vi "Get Menus.vi"(8 "error in (no error)":errorcluster, 9 "Name":string, 10 "RightMenu":refnum<vi>, 11 "Left Menu":refnum<vi>) -> (0 "error out":errorcluster)   [LabVIEW 2020]
doc: "This VI provides access to the defined set of menus, returning whichever is requested by the caller. It provides encapsulation of the menu list, so the list can be updated/modified without having to change this function or its callers."
uses:
  Controls/Menu.ctl
  Controls/Menus.ctl
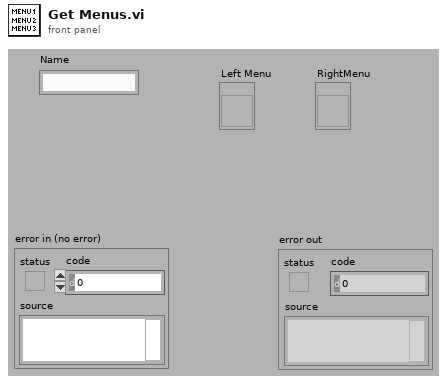
[diagram p1: front panel]
types:
  T1 = typedef "Menus.ctl" = cluster{"Menu Name":string, "Left Menu":T2, "Right Menu":T2}[]
  T2 = typedef "Menu.ctl" = cluster{"Menu 0":string, "Menu 1":string, "Menu 2":string}
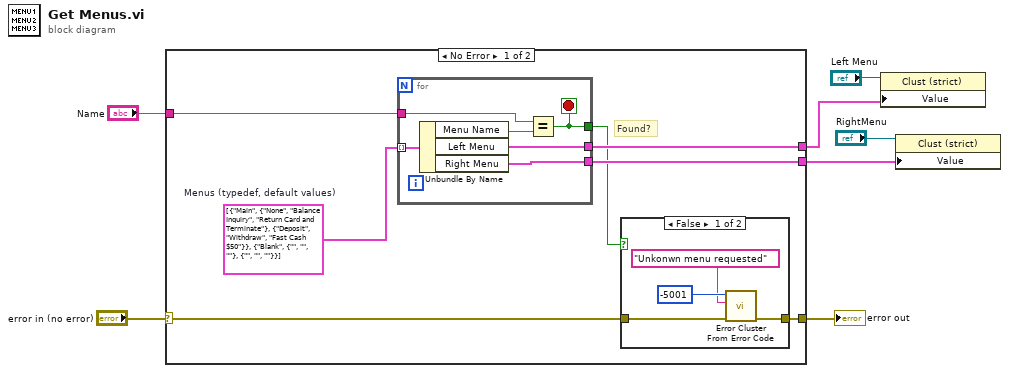
[diagram p0: block diagram]
diagram:
  n1 = case shown="No Error" "error in (no error)" {
    selector: "error in (no error)" -> [w8 w26]
    tunnel: "Name" -> [w14 _]
    tunnel: [w12 _] -> w3
    tunnel: [w11 _] -> w2
    tunnel: [w9 w26] -> w6
    frame No Error {
      w13 = T1 [{"Menu Name"="Main", "Left Menu"={"Menu 0"="None", "Menu 1"="Balance Inquiry", "Menu 2"="Return Card and Terminate"}, "Right Menu"={"Menu 0"="Deposit", "Menu 1"="Withdraw", "Menu 2"="Fast Cash $50"}}, {"Menu Name"="Blank", "Left Menu"={"Menu 0"="", "Menu 1"="", "Menu 2"=""}, "Right Menu"={"Menu 0"="", "Menu 1"="", "Menu 2"=""}}]  # Menus (typedef, default values)
      # "Found?"
      n2 = for {
        tunnel: w13 -> [w25] mode=indexing
        tunnel: w14 -> [w23]
        tunnel: [w22] -> w10
        tunnel: [w21] -> w12
        tunnel: [w20] -> w11
        stop <- w22 stop-if-true
        n3 = Unbundle By Name(w25) -> ("Menu Name"=w24:string, "Left Menu"=w21:T2, "Right Menu"=w20:T2)
        n4 = Equal?(x=w23, y=w24) -> (x = y?=w22:bool)
      }
      n5 = case shown="False" w10 {
        tunnel: w8 -> [w18 w19]
        tunnel: [w17 w19] -> w9
        frame False {
          n6 = call <vilib>:"Error Cluster From Error Code.vi"("error in (no error)"=w18, "error message (\"\")"="Unkonwn menu requested" ("error message (\"\")"), "error code (0)"=-5001) -> ("error out"=w17:errorcluster)  [unwired: 6 in]
        }
        frame True {
        }
      }
    }
    frame Error {
    }
  }
  "error out" <- w6
  n7 = property on="Property Node" class="Clust (strict)"(reference="Left Menu", "Value"=w3) -> ()  [unwired: 1 in, 2 out]
  n8 = property on="Property Node" class="Clust (strict)"(reference="RightMenu", "Value"=w2) -> ()  [unwired: 1 in, 2 out]
